vi "Get-max-clients.vi"(8 "error in (no error)":errorcluster, 10 "Module type":T1=enum."Server", 11 "ModComm in":T2) -> (0 "error out":errorcluster, 2 "Max clients":i32, 3 "ModComm out":T2)   [LabVIEW 2013, in "SLMServer.lvlib" / "SLMServer.lvclass"]
uses:
  SLMServer.lvclass
  Object-reference.ctl
  Supported-module-types.ctl
  SLMServer.lvclass/SLMServer.ctl
  Read Max clients.vi
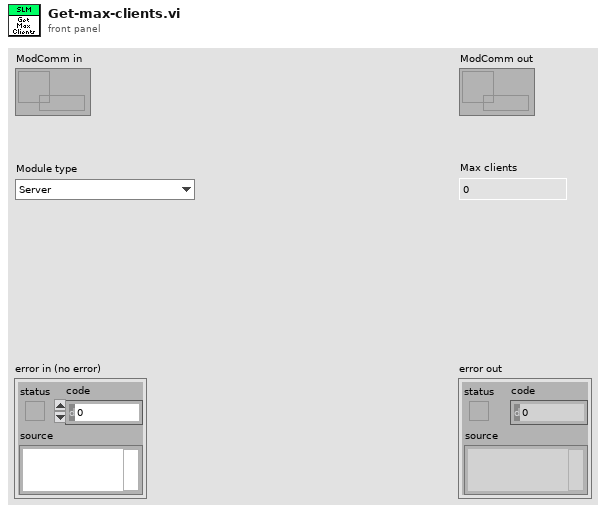
[diagram p1: front panel]
types:
  T1 = typedef "SLMServer.lvlib/SLMServer.lvclass/Supported-module-types.ctl" = enum16{"SLMControl", "PowderDeposition", "CameraVision", "Server", "All", "StrategyParser", "MaterialCharacterization", "StatusMonitor", "SLMSimulation", "LaserCharacterization"}
  T2 = typedef "SLMServer.lvlib/SLMServer.lvclass/Object-reference.ctl" = refnum<data-value>
  T3 = cluster{"Module type":T1, "MaxClients":i32, "Path":path, "Path type":bool}[]
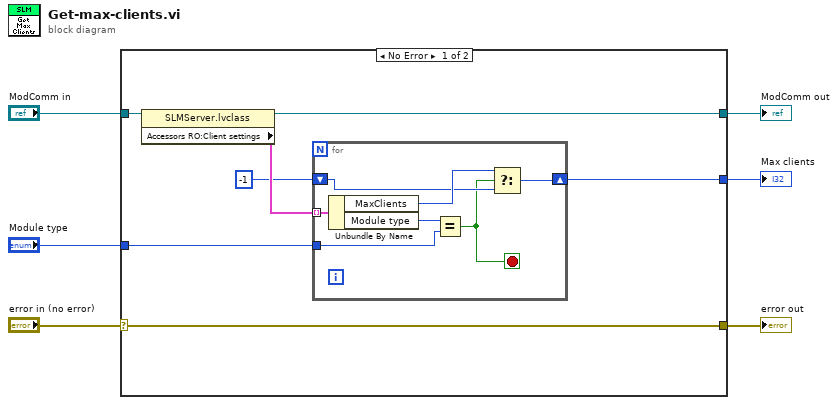
[diagram p0: block diagram]
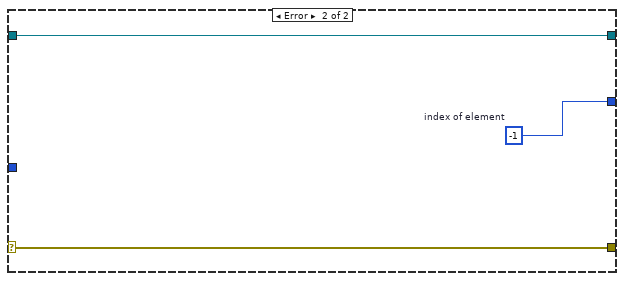
[diagram p2: hidden frame]
diagram:
  n1 = case shown="No Error" "error in (no error)" {
    selector: "error in (no error)" -> [w13 w23]
    tunnel: [w13 w23] -> w5
    tunnel: [w11 w22] -> w3
    tunnel: "ModComm in" -> [w12 w22]
    tunnel: "Module type" -> [w9 _]
    tunnel: [w7 w21] -> w1
    frame No Error {
      n2 = property class="SLMServer.lvclass"(reference=w12) -> (reference out=w11:T2, "Accessors RO:Client settings"=w10:T3)  [unwired: 1 in, 1 out]
      n3 = for {
        tunnel: w10 -> [w20] mode=indexing
        tunnel: w9 -> [w19]
        shift-right: [w16] -> w7
        shift-left: -1 -> [w15]
        stop <- w14 stop-if-true
        n4 = Unbundle By Name(w20) -> ("MaxClients"=w17:i32, "Module type"=w18:T1)
        n5 = Equal?(x=w18, y=w19) -> (x = y?=w14:bool)
        n6 = Select(t=w17, s=w14, f=w15) -> (s? t:f=w16:i32)
      }
    }
    frame Error {
      w21 = -1  # index of element
    }
  }
  "error out" <- w5
  "ModComm out" <- w3
  "Max clients" <- w1
